vi "ln_v2.vi"(8 "ready for output (T)":bool=TRUE, 9 "input valid":bool=TRUE, 10 "x":fxp<+,32,16>) -> (0 "ready for input":bool, 1 "output valid":bool, 2 "ln(x)":fxp<+/-,23,6>)   [LabVIEW 2018]
uses:
  <vilib>/rvi/FXPMathLib/FxpLn/subVIs/nifxpmath_NaturalLogarithm_SimConfig.ctl
  <vilib>/rvi/FXPMathLib/FxpLn/simVIs/DllFxpNaturalLogarithmTemp_sub.vi
  <vilib>/rvi/FXPMathLib/FxpInterpret/XNode/nifxpmath_Interpret.xnode
  <vilib>/rvi/FXPMathLib/FxpLn/XNode/nifxpmath_NaturalLogarithm.xnode
  <vilib>/rvi/FXPMathLib/FxpAdd/XNode/nifxpmath_Add.xnode
  <vilib>/rvi/FXPMathLib/sim/FxpSim.dll
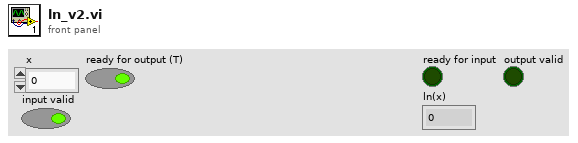
[diagram p1: front panel]
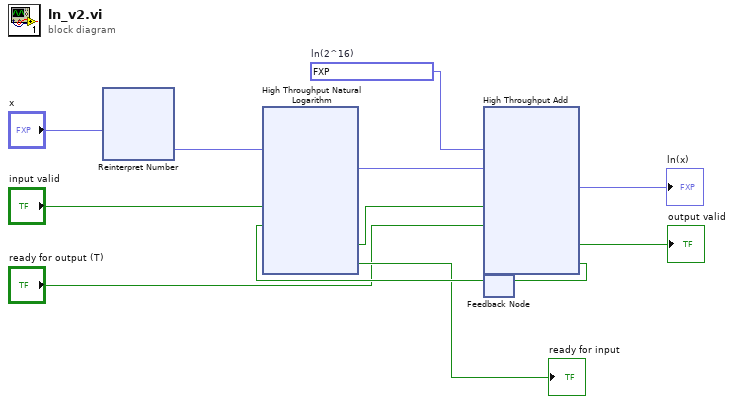
[diagram p0: block diagram]
diagram:
  w8 = fxp<+,21,4> 11.090354919433594  # ln(2^16)
  n1 = xnode "Reinterpret Number"("x"="x") -> ("y"=w11:fxp<+,32,0>)
  n2 = feedback #1() -> (w5:bool)  [unwired: 1 in]
  n3 = xnode "High Throughput Natural Logarithm"("x"=w11, "input valid"="input valid", "ready for output (T)"=w5) -> ("ln(x)"=w9:fxp<+/-,16,1>, "output valid"=w7:bool, "ready for input"=→"ready for input":bool)  [unwired: 1 out]
  n4 = xnode "High Throughput Add"("x"=w8, "y"=w9, "input valid"=w7, "ready for output (T)"="ready for output (T)") -> ("x+y"=→"ln(x)":fxp<+/-,23,6>, "output valid"=→"output valid":bool, "ready for input"=w6:bool)
  n5 = feedback-in #1(w6) -> ()
